vi "GF_UpdateGraphList.vi"(1 "error in (no error)":errorcluster, 2 "Wavenames Array":string[](array[string]), 3 "Graph Ref Array":refnum<vi>[](array[refnum])) -> (0 "error out":errorcluster)   [LabVIEW 2016]
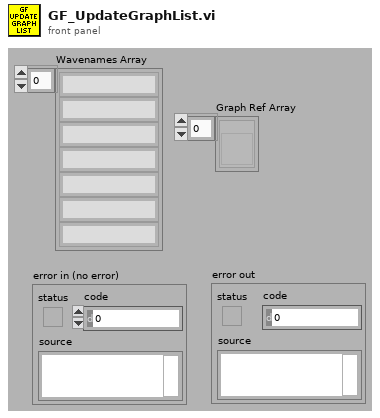
[diagram p1: front panel]
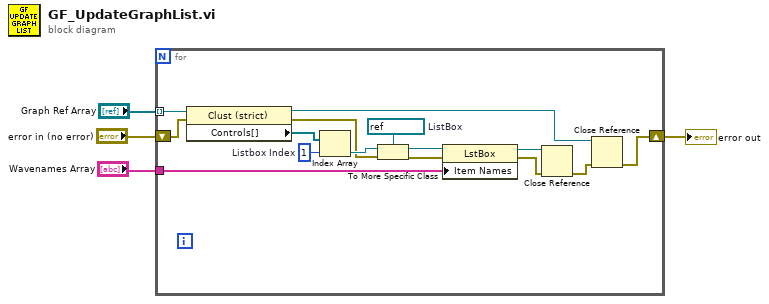
[diagram p0: block diagram]
diagram:
  n1 = for {
    tunnel: "Graph Ref Array" -> [w19] mode=indexing
    tunnel: "Wavenames Array" -> [w14]
    shift-right: [w6] -> w2
    shift-left: "error in (no error)" -> [w5]
    w15 = refnum<vi> refnum  # ListBox
    w17 = 1  # Listbox Index
    n2 = property class="Clust (strict)"(reference=w19, error in=w5) -> (reference out=w7:refnum<vi>, error out=w9:errorcluster, "Controls[]"=w18:refnum<vi>[])
    n3 = Index Array(array=w18, index=w17) -> (element=w16:refnum<vi>)
    n4 = To More Specific Class(target class=w15, reference=w16, error in=w9) -> (specific class reference=w13:refnum<vi>, error out=w10:errorcluster)
    n5 = property class="LstBox"(reference=w13, error in=w10, "Item Names"=w14) -> (reference out=w12:refnum<vi>, error out=w11:errorcluster)
    n6 = Close Reference(reference=w12, error in (no error)=w11) -> (error out=w8:errorcluster)
    n7 = Close Reference(reference=w7, error in (no error)=w8) -> (error out=w6:errorcluster)
  }
  "error out" <- w2
